vi "Actor Core.vi"(8 "error in":errorcluster, 11 "CS++DCPwrGui.lvclass":refnum<class "CS++FgenGui.lvclass">) -> (0 "Error Out":errorcluster, 3 "Actor out":refnum<class "Actor.lvclass">)   [LabVIEW 2015, in "CS++FgenGui.lvlib" / "CS++FgenGui.lvclass"]
doc: "(<B>Filename</B>: Actor Framework.lvlib:Actor.lvclass:Actor Core.vi)\n\nReceives messages to the actor, reacts to them, and initiates any error handling that may shut the actor down.\n\nDescendant classes may override this VI to append parallel tasks for the actor to complete while it handles messages. Overrides use the Call Parent Method node."
uses:
  CS++FgenGui.lvclass
  <vilib>/ActorFramework/Actor/Actor.lvclass
  CSPP_Core/Actors/CS++BaseActor/CS++BaseActor.lvclass/CS++BaseActor.ctl
  CSPP_Core/Actors/CS++GUIActor/CS++GUIActor.lvclass/CS++GUIActor.ctl
  CS++FgenChannelData/CS++FgenChannelData.lvclass
  <vilib>/ActorFramework/Actor/Actor.lvclass/Actor.ctl
  <vilib>/ActorFramework/Message Enqueuer/Message Enqueuer.lvclass/Message Enqueuer.ctl
  CSPP_Core/Classes/CS++ProcessVariables/ProcessVariable/PV.lvclass/PV.ctl
  CS++FgenChannelData/CS++FgenChannelData.lvclass/CS++FgenChannelData.ctl
  CSPP_Core/Actors/CS++BaseActor/Read Object Name.vi
  CSPP_Core/Actors/CS++BaseActor/Read CS++Factory.vi
  CSPP_Core/Actors/CS++GUIActor/Read Associated Actor Name.vi
  CSPP_Core/Classes/CS++ProcessVariables/ProcessVariable/Read Data.vi
  CSPP_Core/Classes/CS++ProcessVariables/ProcessVariable/Read Timestamp.vi
  CSPP_Core/Classes/CS++ProcessVariables/ProcessVariable/Read Name.vi
  CSPP_Core/Actors/CS++GUIActor/Read Stop-Event.vi
  CSPP_Core/Actors/CS++GUIActor/Read PV-Update.vi
  <vilib>/ActorFramework/Message Enqueuer/Init from Existing Queue.vi
  <vilib>/ActorFramework/Message Enqueuer/Enqueue.vi
  <vilib>/ActorFramework/Message Priority Queue/Priority Enqueue.vi
  CSPP_Core/Classes/CS++ProcessVariables/PVConnection/PVConnection.lvclass
  CSPP_Core/Classes/CS++BaseClasses/Factory/CS++Factory.lvclass
  CSPP_Core/Classes/CS++ProcessVariables/ProcessVariable/PV.lvclass
  <vilib>/ActorFramework/Message Enqueuer/Message Enqueuer.lvclass
  <vilib>/ActorFramework/Stop Msg/Stop Msg.lvclass
  CSPP_Core/Actors/CS++DeviceGUIActor/CS++DeviceGUIActor.lvclass
  CSPP_Core/Actors/CS++BaseActor/CS++BaseActor.lvclass
  CSPP_Core/Libraries/Utilities/CS++Utilities.lvlib
  CSPP_Core/Actors/CS++GUIActor/CS++GUIActor.lvclass
panel:
  in  "Tab Control":T1(tab)
  out "Associated Device Actor":string
  out "Driver Revision":string
  out "Firmware Revision":string
  out "Self-Test Result Code":i32
  out "Self-Test Result Message":string
  out "Resource Name":string
  out "Number Of Channels":i32
  out "Timestamp":timestamp
  in  "Tab Control 2":enum32{"General", "Channel"}(tab)
  in  "Sample Clock Output Enabled (Disabled)":bool caption="Sample Clock Output Enabled"
  in  "Sample Rate (1000 Samp/s)":dbl[unit]=1000.0 caption="Sample Rate" format="%.3e"
  in  "Internal Trigger Rate":dbl[unit] format="%^.3e"
  in  "Output Mode":i32(ring) items=["Standard Function", "Arbitrary Waveform", "Arbitrary Sequence"]
  in  "Reference Clock Source":i32(ring) caption="reference clock source (Internal)" items=["Internal"=0, "External"=1, "RTSI Clock"=101]
  in  "Sample Clock Source (Internal)":i32(ring) caption="Sample Clock Source" items=["Internal", "External"]
  in  "Config AM Modulation":bool
  in  "modulation frequency (1000 Hz)":dbl[unit]=1000.0 caption="AM Modulation Frequency" format="%^.2e"
  in  "modulation depth (0.00 %)":dbl caption="AM Modulation Depth /%" format="%.3f"
  in  "AM Modulation Waveform":i32(ring)=1 caption="modulation waveform (Sine)" items=["Sine"=1, "Square"=2, "Triangle"=3, "Ramp Up"=4, "Ramp Down"=5]
  in  "Config FM Modulation":bool
  in  "FM Modulation Frequency (1000 Hz)":dbl[unit]=1000.0 caption="FM Modulation Frequency" format="%^.2e"
  in  "FM Peak Deviation":dbl[unit]=100.0 format="%^.2e"
  in  "FM Modulation Waveform":i32(ring)=1 items=["Sine"=1, "Square"=2, "Triangle"=3, "Ramp Up"=4, "Ramp Down"=5]
  in  "Channel Index":i32 min=0 max=0 step=1
  in  "Tab Control 3":T2(tab)
  in  "Standard-Waveform":T3={"Enabled"=TRUE, "Operation Mode"=0, "Impedance"=50.0, "Waveform"=1, "Frequency"=1000.0, "Amplitude"=1.0, "DC Offset"=0.0, "Trigger Source"=1, "Burst Count"=1, "Start Phase"=0.0, "Set/Single"=FALSE} {"Start Phase" format="%.3f"; "Trigger Source" items=["Internal"=3, "External"=1, "Software Trigger Function"=2, "PXI TRIG0 or VXI TTL0"=111, "PXI TRIG1 or VXI TTL1"=112, "PXI TRIG2 or VXI TTL2"=113, "PXI TRIG3 or VXI TTL3"=114, "PXI TRIG4 or VXI TTL4"=115, "PXI TRIG5 or VXI TTL5"=116, "PXI TRIG6 or VXI TTL6"=117, "PXI TRIG7 or VXI TTL7"=118, "ECL0"=119, "ECL1"=120, "PXI Star"=131, "RTSI 0"=141, "RTSI 1"=142, "RTSI 2"=143, "RTSI 3"=144, "RTSI 4"=145, "RTSI 5"=146, "RTSI 6"=147]; "Frequency" format="%^.3e"; "DC Offset" format="%.3f"; "Amplitude" format="%.3f"; "Waveform" items=["Sine"=1, "Square"=2, "Triangle"=3, "Ramp Up"=4, "Ramp Down"=5, "DC"=6]; "Impedance" format="%.3f"; "Operation Mode" items=["Continuous", "Burst"]}
  in  "AM-Modulation":cluster{"Enabled":bool, "Source":i32}={"Enabled"=TRUE, "Source"=0} {"Source" items=["Internal", "External"]}
  in  "FM-Modulation":cluster{"Enabled":bool, "Source":i32}={"Enabled"=TRUE, "Source"=0} {"Source" items=["Internal", "External"]}
  in  "Advanced Trigger":T4 {"Trigger Slope)" items=["Positive", "Negative", "Either"]}
  in  "Start Trigger":T5 {"Trigger Slope" items=["Positive", "Negative", "Either"]}
  in  "Stop Trigger":T4 {"Trigger Slope)" items=["Positive", "Negative", "Either"]}
  in  "Resume Trigger":T4 {"Trigger Slope)" items=["Positive", "Negative", "Either"]}
  in  "Clear Arbitrary Waveform":bool
  in  "Clear Arbitrary Sequence":bool
  in  "Clear Arbitrary Memory":bool
  in  "SW Trigger":bool
  in  "SW Stop Trigger":bool
  in  "SW Resume Trigger":bool
  in  "SW Hold Trigger":bool
  in  "SW Advanced Trigger":bool
  in  "Initiate Generation":bool
  in  "Abort Generation":bool
  in  "Stop Button":bool
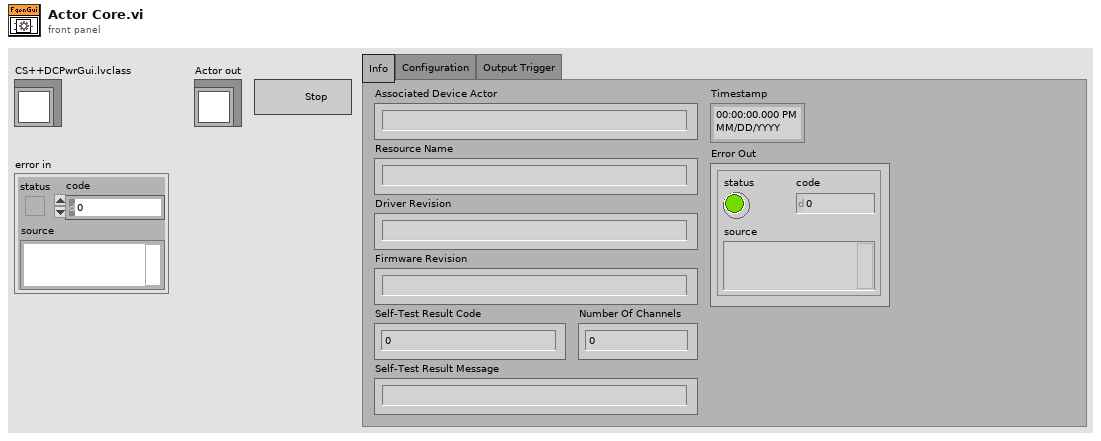
[diagram p1: front panel]
types:
  T1 = enum32{"Info", "Configuration", "Output Trigger"}
  T2 = enum32{"General", "AM/FM-Modulation", "More Trigger"}
  T3 = cluster{"Enabled":bool, "Operation Mode":i32, "Impedance":dbl[unit], "Waveform":i32, "Frequency":dbl[unit], "Amplitude":dbl[unit], "DC Offset":dbl[unit], "Trigger Source":i32, "Burst Count":i32, "Start Phase":dbl[unit], "Set/Single":bool}
  T4 = cluster{"Trigger Source":string, "Trigger Slope)":i32}
  T5 = cluster{"Trigger Source":string, "Trigger Slope":i32}
  T6 = enum32{"Invalid", "Standard", "Closed", "Hidden", "Minimized", "Maximized"}
  T7 = cluster{"AM Modulation Waveform":i32, "modulation depth (0.00 %)":dbl, "modulation frequency (1000 Hz)":dbl[unit]}
  T8 = cluster{"FM Modulation Waveform":i32, "FM Peak Deviation":dbl[unit], "FM Modulation Frequency (1000 Hz)":dbl[unit]}
  T9 = cluster{"Trigger Slope":i32, "Substring":string, "Trigger Source":string}
  T10 = cluster{"Trigger Slope)":i32, "Substring":string, "Trigger Source":string}
  T11 = cluster{"Start Phase":dbl[unit], "Frequency":dbl[unit], "DC Offset":dbl[unit], "Substring":string, "Amplitude":dbl[unit], "Waveform":i32}
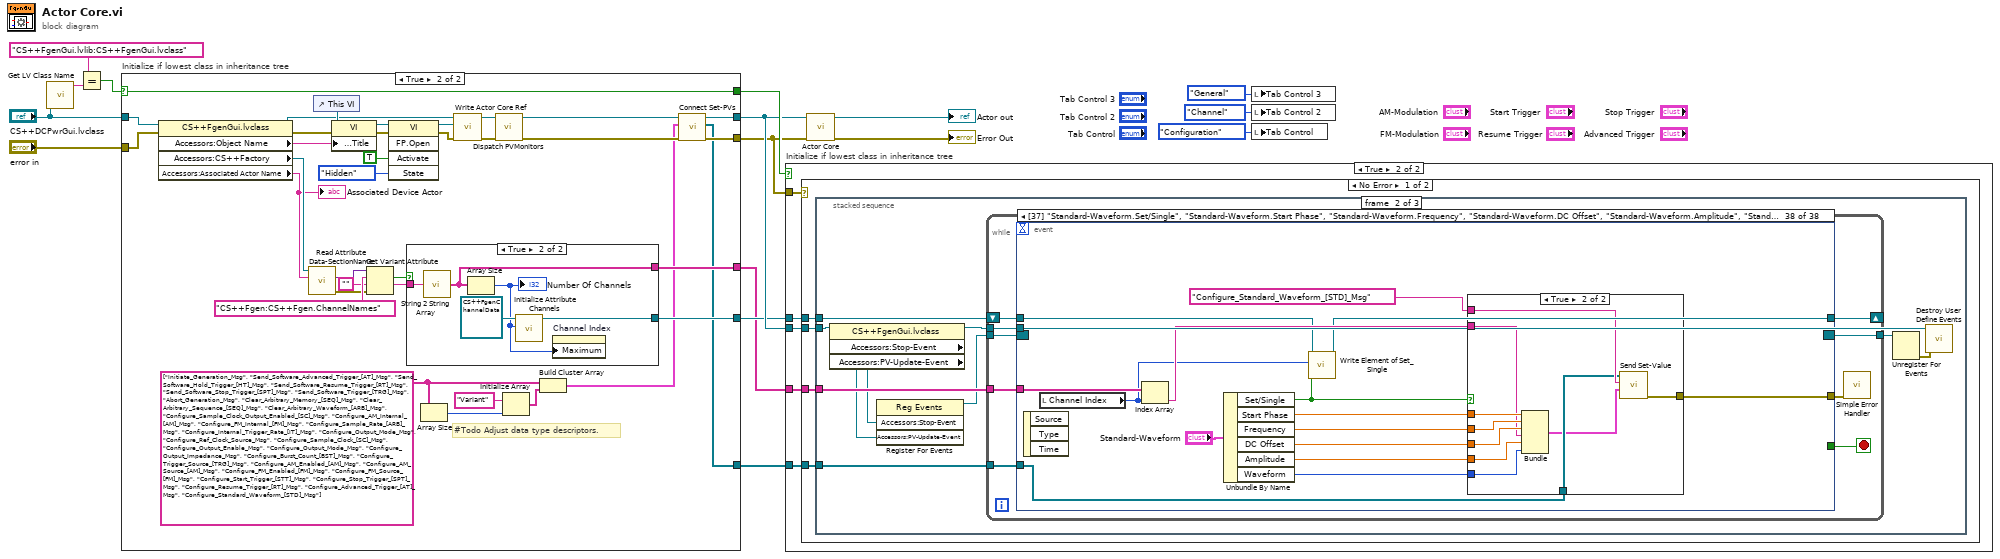
[diagram p0: block diagram]
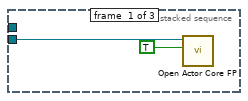
[diagram p5: hidden frame]
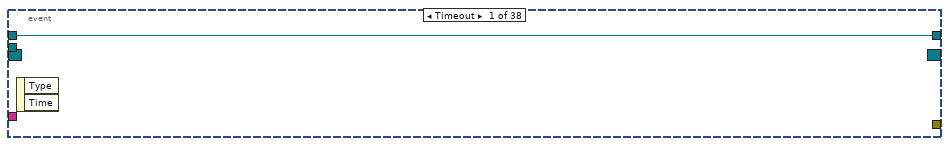
[diagram p6: hidden frame]
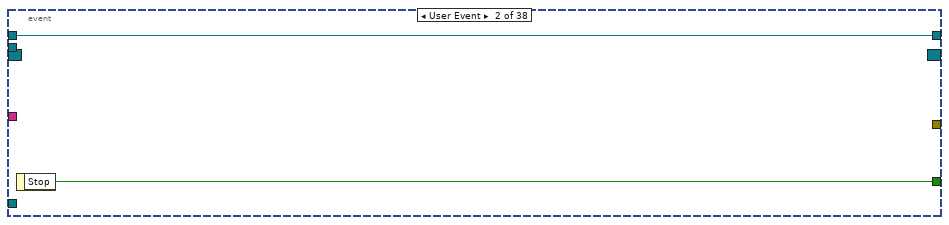
[diagram p7: hidden frame]
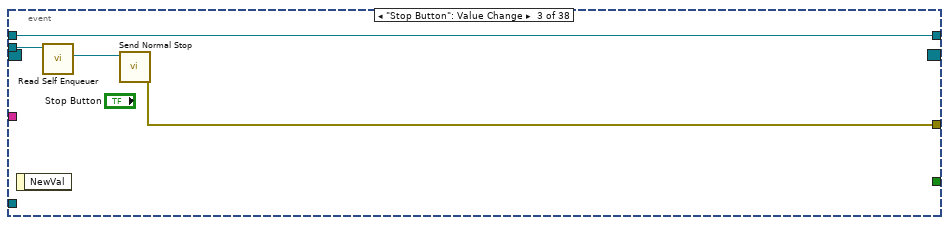
[diagram p8: hidden frame]
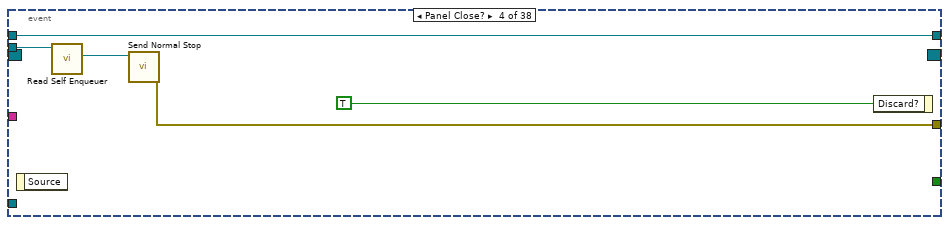
[diagram p9: hidden frame]
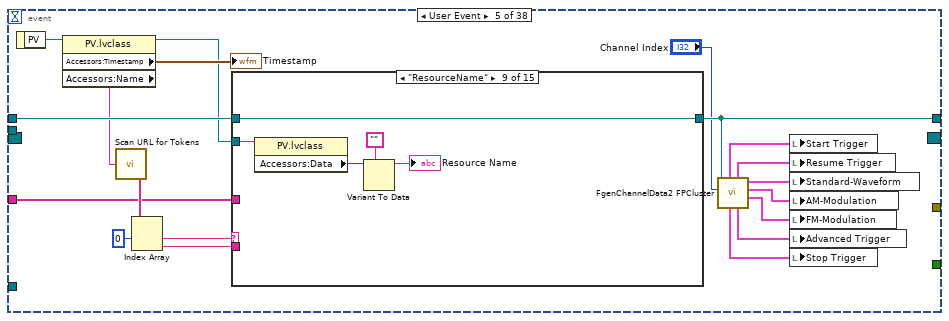
[diagram p10: hidden frame]
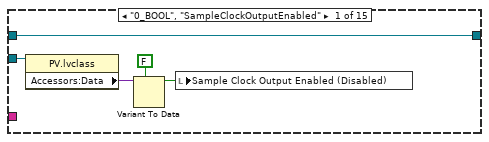
[diagram p11: hidden frame]
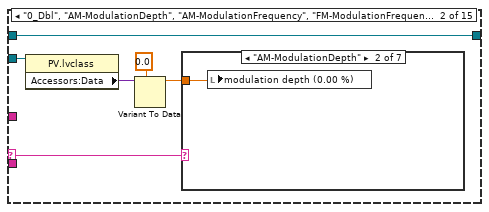
[diagram p12: hidden frame]
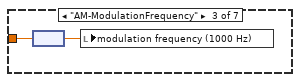
[diagram p14: hidden frame]
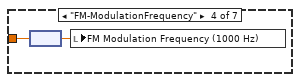
[diagram p15: hidden frame]
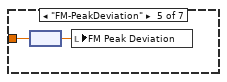
[diagram p16: hidden frame]
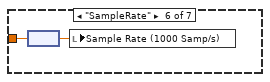
[diagram p17: hidden frame]
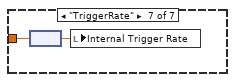
[diagram p18: hidden frame]
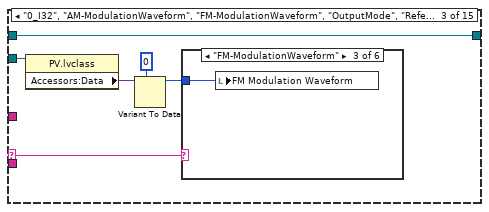
[diagram p19: hidden frame]
diagram:
  n1 = call <vilib>:"Get LV Class Name.vi"("object"="CS++DCPwrGui.lvclass") -> ("class name"=w14:string)  [unwired: 9 in, 1 out]
  n2 = Equal?(x="CS++FgenGui.lvlib:CS++FgenGui.lvclass" ("class name"), y=w14) -> (x = y?=w12:bool)
  n3 = case "Initialize if lowest class in inheritance tree" shown="True" w12 {
    selector: w12 -> [w17 w54]
    tunnel: [w18 w28] -> w7
    tunnel: "error in" -> [w18 w34]
    tunnel: [w19 w26] -> w8
    tunnel: "CS++DCPwrGui.lvclass" -> [w19 w35]
    tunnel: [w17 w54] -> w11
    tunnel: [_ w49] -> w6
    tunnel: [_ w48] -> w2
    tunnel: [_ w25] -> w1
    frame False {
    }
    frame True {
      w23 = string[] ["Initiate_Generation_Msg", "Send_Software_Advanced_Trigger_[AT]_Msg", "Send_Software_Hold_Trigger_[HT]_Msg", "Send_Software_Resume_Trigger_[RT]_Msg", "Send_Software_Stop_Trigger_[SPT]_Msg", "Send_Software_Trigger_[TRG]_Msg", "Abort_Generation_Msg", "Clear_Arbitrary_Memory_[SEQ]_Msg", "Clear_Arbitrary_Sequence_[SEQ]_Msg", "Clear_Arbitrary_Waveform_[ARB]_Msg", "Configure_Sample_Clock_Output_Enabled_[SC]_Msg", "Configure_AM_Internal_[AM]_Msg", "Configure_FM_Internal_[FM]_Msg", "Configure_Sample_Rate_[ARB]_Msg", "Configure_Internal_Trigger_Rate_[IT]_Msg", "Configure_Output_Mode_Msg", "Configure_Ref_Clock_Source_Msg", "Configure_Sample_Clock_[SC]_Msg", "Configure_Output_Enable_Msg", "Configure_Output_Mode_Msg", "Configure_Output_Impedance_Msg", "Configure_Burst_Count_[BST]_Msg", "Configure_Trigger_Source_[TRG]_Msg", "Configure_AM_Enabled_[AM]_Msg", "Configure_AM_Source_[AM]_Msg", "Configure_FM_Enabled_[FM]_Msg", "Configure_FM_Source_[FM]_Msg", "Configure_Start_Trigger_[STT]_Msg", "Configure_Stop_Trigger_[SPT]_Msg", "Configure_Resume_Trigger_[RT]_Msg", "Configure_Advanced_Trigger_[AT]_Msg", "Configure_Standard_Waveform_[STD]_Msg"]
      # "#Todo Adjust data type descriptors."
      n4 = property class="CS++FgenGui.lvclass"(reference=w35, error in=w34) -> (reference out=w39:refnum<class "CS++FgenGui.lvclass">, error out=w40:errorcluster, "Accessors:Object Name"=w38:string, "Accessors:CS++Factory"=w31:refnum<class "CS++Factory.lvclass">, "Accessors:Associated Actor Name"=w30:string)
      "Associated Device Actor" <- w30
      n5 = call-dynamic "Read Attribute Data-SectionName.vi"("Object Name"=w30, "CS++Factory in"=w31) -> ("error out"=w32:errorcluster, "Attribute Data"=w33:variant)  [unwired: 7 in, 1 out]
      n6 = control-ref of="This VI"() -> (w43:refnum<vi>)
      n7 = property class="VI"(reference=w43, error in=w40, "Front Panel.Title"=w38) -> (reference out=w42:refnum<vi>, error out=w41:errorcluster)
      n8 = Get Variant Attribute(Variant=w33, name="CS++Fgen:CS++Fgen.ChannelNames", default value (empty Variant)="", error in=w32) -> (found=w51:bool, value=w50:string)  [unwired: 2 out]
      n9 = invoke class="VI" method="FP.Open"(reference=w42, error in=w41, "Activate"=TRUE ("Activate?"), "State"=T6."Hidden") -> (reference out=w45:refnum<vi>, error out=w44:errorcluster)  [unwired: 1 in, 3 out]
      n10 = case shown="True" w51 {
        tunnel: w50 -> [_ w56]
        tunnel: [_ w58] -> w49
        tunnel: [_ w55] -> w48
        frame False {
        }
        frame True {
          n11 = call "String 2 String Array.vi"("String"=w56) -> ("Substrings"=w55:string[])  [unwired: 1 in]
          n12 = Array Size(array=w55) -> (size(s)=w57:i32)
          "Number Of Channels" <- w57
          n13 = call "Initialize Attribute Channels.vi"("Number of Channels"=w57, "CS++FgenChannelData in"=refnum<class "CS++FgenChannelData.lvclass"> refnum ("CS++FgenGui.lvlib:CS++FgenChannelData.lvclass")) -> ("CS++FgenChannelData out"=w58:refnum<class "CS++FgenChannelData.lvclass">)  [unwired: 8 in, 1 out]
          n14 = property on="Channel Index" class="DigNum (strict)"("Maximum"=w57) -> ()  [unwired: 2 in, 2 out]
        }
      }
      n15 = Array Size(array=w23) -> (size(s)=w22:i32)
      n16 = call "Write Actor Core Ref.vi"("error in (no error)"=w44, "Actor Core Ref"=w45, "CS++BaseActor in"=w39) -> ("error out"=w36:errorcluster, "CS++BaseActor out"=w37:refnum<class "CS++FgenGui.lvclass">)  [unwired: 7 in]
      n17 = call "Dispatch PVMonitors.vi"("Error In"=w36, "CS++GUIActor in"=w37) -> ("Error Out"=w29:errorcluster, "CS++GUIActor out"=w27:refnum<class "CS++FgenGui.lvclass">)  [unwired: 8 in]
      n18 = Initialize Array("Variant" ("element"), w22) -> (w20:string[])
      n19 = Build Cluster Array(w23, w20) -> (w24:cluster{string, "element":string}[])
      n20 = call "Connect Set-PVs.vi"("Error In"=w29, "Set-Messages"=w24, "CS++GUIActor in"=w27) -> ("Error Out"=w28:errorcluster, "PVConnections"=w25:refnum<class "PVConnection.lvclass">[], "CS++GUIActor out"=w26:refnum<class "CS++FgenGui.lvclass">)  [unwired: 6 in]
    }
  }
  n21 = case "Initialize if lowest class in inheritance tree" shown="True" w11 {
    tunnel: w7 -> [_ w64]
    tunnel: w8 -> [_ w63]
    tunnel: w6 -> [_ w62]
    tunnel: w2 -> [_ w61]
    tunnel: w1 -> [_ w60]
    frame False {
    }
    frame True {
      n22 = case shown="No Error" w64 {
        tunnel: w63 -> [w68 _]
        tunnel: w62 -> [w67 _]
        tunnel: w61 -> [w66 _]
        tunnel: w60 -> [w65 _]
        frame No Error {
          n23 = stacked-sequence {
            tunnel: w68 -> [w70 w76 w622]
            tunnel: w67 -> [_ w80 _]
            tunnel: w66 -> [_ w79 _]
            tunnel: w65 -> [_ w71 w620]
            frame #0 {
              n24 = call "Open Actor Core FP.vi"("Open FP (F)"=TRUE, "CS++BaseActor in"=w70) -> ()  [unwired: 8 in, 2 out]
            }
            frame #1 {
              n25 = property class="CS++FgenGui.lvclass"(reference=w76) -> (reference out=w75:refnum<class "CS++FgenGui.lvclass">, "Accessors:Stop-Event"=w73:refnum<user-event>, "Accessors:PV-Update-Event"=w72:refnum<user-event>)  [unwired: 1 in, 1 out]
              n26 = register-events(w73, w72) -> (reference out=w74:refnum<event-registration>)  [unwired: 2 in, 1 out]
              n27 = while {
                tunnel: w74 -> [w89]
                tunnel: w75 -> [w88]
                tunnel: [w86] -> w78
                shift-right: [w83] -> _
                shift-left: w80 -> [w84]
                tunnel: w79 -> [w82]
                tunnel: w71 -> [w81]
                stop <- w87 stop-if-true
                n28 = event shown="[37] \"Standard-Waveform.Set/Single\", \"Standard-Waveform.Start Phase\", \"Standard-Waveform.Frequency\", \"Standard-Waveform.DC Offset\", \"Standard-Waveform.Amplitude\", \"Standard-Waveform.Waveform\": Value Change" {
                  selector: w89 -> [_ _ _ _ _ _ _ _ _ _ _ _ _ _ _ _ _ _ _ _ _ _ _ _ _ _ _ _ _ _ _ _ _ _ _ _ _ _]
                  dyn-events: [_ _ _ _ _ _ _ _ _ _ _ _ _ _ _ _ _ _ _ _ _ _ _ _ _ _ _ _ _ _ _ _ _ _ _ _ _ _] -> w86
                  timeout: _ -> [_ _ _ _ _ _ _ _ _ _ _ _ _ _ _ _ _ _ _ _ _ _ _ _ _ _ _ _ _ _ _ _ _ _ _ _ _ _]
                  tunnel: w88 -> [_ _ w96 w99 _ _ _ _ _ _ _ _ _ _ _ _ _ _ _ _ _ _ _ _ _ _ _ _ _ _ _ _ _ _ _ _ _ _]
                  tunnel: [_ w92 _ _ _ _ _ _ _ _ _ _ _ _ _ _ _ _ _ _ _ _ _ _ _ _ _ _ _ _ _ _ _ _ _ _ _ _] -> w87
                  tunnel: [_ _ w94 w98 _ w336 w347 w355 w363 w371 w379 w387 w395 w403 w411 w419 w424 w429 w441 w447 w453 w458 w463 w468 w475 w484 w493 w502 w511 w520 w529 w538 w547 w557 w568 w579 w590 w607] -> w85
                  tunnel: w84 -> [w90 w91 w93 w97 w114 w342 w345 w353 w361 w369 w377 w385 w393 w401 w409 w417 w428 w436 w444 w449 w454 w459 w464 w469 w478 w487 w496 w505 w514 w523 w532 w541 w550 w561 w572 w583 w594 w600]
                  tunnel: [w90 w91 w93 w97 w106 w342 w345 w353 w361 w369 w377 w385 w393 w401 w409 w417 w428 w436 w444 w449 w454 w459 w464 w469 w478 w487 w496 w505 w514 w523 w532 w541 w550 w561 w572 w583 w594 w599] -> w83
                  tunnel: w82 -> [_ _ _ _ w104 _ _ _ _ _ _ _ _ _ _ _ _ _ _ _ _ _ _ _ w477 w486 w495 w504 w513 w522 w531 w540 w549 w560 w571 w582 w593 w609]
                  tunnel: w81 -> [_ _ _ _ _ _ w344 w352 w360 w368 w376 w384 w392 w400 w408 w416 w426 w434 w442 w446 w452 w456 w461 w466 w473 w483 w491 w500 w510 w519 w527 w536 w546 w555 w567 w578 w588 w595]
                  event Timeout {
                    n29 = event-data() -> ()  [unwired: 1 in, 2 out]
                  }
                  event User Event {
                    n30 = event-data() -> ("Stop"=w92:bool)  [unwired: 1 in]
                  }
                  event "Stop Button": Value Change {
                    n31 = event-data() -> ()  [unwired: 1 in, 1 out]
                    n32 = call <vilib>:"Read Self Enqueuer.vi"("Actor"=w96) -> ("Self Enqueuer"=w95:refnum<class "Message Enqueuer.lvclass">)  [unwired: 10 in]
                    n33 = call <vilib>:"Send Normal Stop.vi"("Message Enqueuer"=w95) -> ("error out"=w94:errorcluster)  [unwired: 10 in]
                  }
                  event Panel Close? {
                    n34 = event-data() -> ()  [unwired: 1 in, 1 out]
                    n35 = call <vilib>:"Read Self Enqueuer.vi"("Actor"=w99) -> ("Self Enqueuer"=w100:refnum<class "Message Enqueuer.lvclass">)  [unwired: 10 in]
                    n36 = call <vilib>:"Send Normal Stop.vi"("Message Enqueuer"=w100) -> ("error out"=w98:errorcluster)  [unwired: 10 in]
                    n37 = event-data("Discard?"=TRUE) -> ()  [unwired: 1 in, 1 out]
                  }
                  event User Event {
                    n38 = event-data() -> ("PV"=w117:refnum<class "PV.lvclass">)  [unwired: 1 in]
                    n39 = property class="PV.lvclass"(reference=w117) -> (reference out=w102:refnum<class "PV.lvclass">, "Accessors:Timestamp"=→"Timestamp":timestamp, "Accessors:Name"=w103:string)  [unwired: 1 in, 1 out]
                    n40 = call "Scan URL for Tokens.vi"("URL"=w103) -> ("Tokens"=w120:string[])
                    n41 = Index Array(array=w120, index #1=0 ("index")) -> (element #1=w115:string, element #2=w118:string)  [unwired: 1 in]
                    n42 = case shown="\"ResourceName\"" w115 {
                      selector: w115 -> [_ w128 w145 w160 w183 w234 w275 _ _ _ _ _ _ _ _]
                      tunnel: w102 -> [w125 w129 w146 w161 w184 w235 w277 _ w298 w303 w308 w314 w319 w324 w330]
                      tunnel: w118 -> [_ _ _ w155 w178 w229 w270 _ _ _ _ _ _ _ _]
                      tunnel: [w121 w126 w143 w159 w182 w233 w274 w296 w301 w306 w311 w317 w322 w327 w333] -> w106
                      tunnel: w114 -> [w121 w126 w143 w158 w181 w232 w273 w296 w301 w306 w311 w317 w322 w327 w333]
                      tunnel: w104 -> [_ _ _ w156 w179 w230 w271 _ _ _ _ _ _ _ _]
                      frame "0_BOOL", "SampleClockOutputEnabled" {
                        n43 = property class="PV.lvclass"(reference=w125) -> ("Accessors:Data"=w123:variant)  [unwired: 1 in, 2 out]
                        n44 = Variant To Data(type=FALSE, Variant=w123) -> (data=w122:bool)  [unwired: 1 in, 1 out]
                        n45 = local write "Sample Clock Output Enabled (Disabled)"(w122) -> ()
                      }
                      frame "0_Dbl", "AM-ModulationDepth", "AM-ModulationFrequency", "FM-ModulationFrequency", "FM-PeakDeviation", "SampleRate", "TriggerRate" {
                        n46 = property class="PV.lvclass"(reference=w129) -> ("Accessors:Data"=w130:variant)  [unwired: 1 in, 2 out]
                        n47 = Variant To Data(type=0.0, Variant=w130) -> (data=w127:dbl)  [unwired: 1 in, 1 out]
                        n48 = case shown="\"AM-ModulationDepth\"" w128 {
                          tunnel: w127 -> [_ w132 w134 w136 w138 w140 w142]
                          frame Default {
                          }
                          frame "AM-ModulationDepth" {
                            n49 = local write "modulation depth (0.00 %)"(w132) -> ()
                          }
                          frame "AM-ModulationFrequency" {
                            n50 = node(w134) -> (w133:dbl[unit])
                            n51 = local write "modulation frequency (1000 Hz)"(w133) -> ()
                          }
                          frame "FM-ModulationFrequency" {
                            n52 = node(w136) -> (w135:dbl[unit])
                            n53 = local write "FM Modulation Frequency (1000 Hz)"(w135) -> ()
                          }
                          frame "FM-PeakDeviation" {
                            n54 = node(w138) -> (w137:dbl[unit])
                            n55 = local write "FM Peak Deviation"(w137) -> ()
                          }
                          frame "SampleRate" {
                            n56 = node(w140) -> (w139:dbl[unit])
                            n57 = local write "Sample Rate (1000 Samp/s)"(w139) -> ()
                          }
                          frame "TriggerRate" {
                            n58 = node(w142) -> (w141:dbl[unit])
                            n59 = local write "Internal Trigger Rate"(w141) -> ()
                          }
                        }
                      }
                      frame "0_I32", "AM-ModulationWaveform", "FM-ModulationWaveform", "OutputMode", "ReferenceClockSource", "SampleClockSource" {
                        n60 = property class="PV.lvclass"(reference=w146) -> ("Accessors:Data"=w147:variant)  [unwired: 1 in, 2 out]
                        n61 = Variant To Data(type=0, Variant=w147) -> (data=w144:i32)  [unwired: 1 in, 1 out]
                        n62 = case shown="\"FM-ModulationWaveform\"" w145 {
                          tunnel: w144 -> [_ w149 w150 w151 w152 w153]
                          frame Default {
                          }
                          frame "AM-ModulationWaveform" {
                            n63 = local write "AM Modulation Waveform"(w149) -> ()
                          }
                          frame "FM-ModulationWaveform" {
                            n64 = local write "FM Modulation Waveform"(w150) -> ()
                          }
                          frame "OutputMode" {
                            n65 = local write "Output Mode"(w151) -> ()
                          }
                          frame "ReferenceClockSource" {
                            n66 = local write "Reference Clock Source"(w152) -> ()
                          }
                          frame "SampleClockSource" {
                            n67 = local write "Sample Clock Source (Internal)"(w153) -> ()
                          }
                        }
                      }
                      frame "0_[Bool]", "AM-Enabled", "ChannelEnabled", "FM-Enabled" {
                        n68 = property class="PV.lvclass"(reference=w161) -> ("Accessors:Data"=w162:variant)  [unwired: 1 in, 2 out]
                        n69 = Search 1D Array(1D array=w156, element=w155) -> (index of element=w154:i32)  [unwired: 1 in]
                        n70 = Variant To Data(type=FALSE, Variant=w162) -> (data=w157:bool)  [unwired: 1 in, 1 out]
                        n71 = case shown="\"AM-Enabled\"" w160 {
                          tunnel: [w164 w167 w171 w175] -> w159
                          tunnel: w158 -> [w164 w168 w172 w176]
                          tunnel: w154 -> [_ w166 w170 w173]
                          tunnel: w157 -> [_ w165 w169 w174]
                          frame Default {
                          }
                          frame "AM-Enabled" {
                            n72 = call "Write Element of AM Enabled.vi"("AM enabled (True)"=w165, "index"=w166, "CS++FgenChannelData in"=w168) -> ("CS++FgenChannelData out"=w167:refnum<class "CS++FgenChannelData.lvclass">)  [unwired: 7 in, 1 out]
                          }
                          frame "ChannelEnabled" {
                            n73 = call "Write Element of Channel Enabled.vi"("channel enabled (True)"=w169, "index"=w170, "CS++FgenChannelData in"=w172) -> ("CS++FgenChannelData out"=w171:refnum<class "CS++FgenChannelData.lvclass">)  [unwired: 7 in, 1 out]
                          }
                          frame "FM-Enabled" {
                            n74 = call "Write Element of FM enabled.vi"("FM enabled (True)"=w174, "index"=w173, "CS++FgenChannelData in"=w176) -> ("CS++FgenChannelData out"=w175:refnum<class "CS++FgenChannelData.lvclass">)  [unwired: 7 in, 1 out]
                          }
                        }
                      }
                      frame "0_[I32]", "AM-Source", "AdvancedTriggerSlope", "BurstCount", "FM-Source", "OperationMode", "ResumeTriggerSlope", "StartTriggerSlope", "StopTriggerSlope", "TriggerSource", "Waveform" {
                        n75 = property class="PV.lvclass"(reference=w184) -> ("Accessors:Data"=w185:variant)  [unwired: 1 in, 2 out]
                        n76 = Search 1D Array(1D array=w179, element=w178) -> (index of element=w177:i32)  [unwired: 1 in]
                        n77 = Variant To Data(type=0, Variant=w185) -> (data=w180:i32)  [unwired: 1 in, 1 out]
                        n78 = case shown="\"AM-Source\"" w183 {
                          tunnel: [w187 w188 w194 w198 w202 w206 w208 w214 w218 w222 w226] -> w182
                          tunnel: w181 -> [w187 w191 w195 w199 w203 w207 w211 w215 w219 w223 w227]
                          tunnel: w177 -> [_ w190 w193 w197 w201 w204 w209 w213 w217 w221 w225]
                          tunnel: w180 -> [_ w189 w192 w196 w200 w205 w210 w212 w216 w220 w224]
                          frame Default {
                          }
                          frame "AM-Source" {
                            n79 = call "Write Element of AM Source.vi"("source (Internal)"=w189, "index"=w190, "CS++FgenChannelData in"=w191) -> ("CS++FgenChannelData out"=w188:refnum<class "CS++FgenChannelData.lvclass">)  [unwired: 7 in, 1 out]
                          }
                          frame "AdvancedTriggerSlope" {
                            n80 = call "Write Element of Advanced Trigger Slope.vi"("Trigger Slope (Positive)"=w192, "index"=w193, "CS++FgenChannelData in"=w195) -> ("CS++FgenChannelData out"=w194:refnum<class "CS++FgenChannelData.lvclass">)  [unwired: 7 in, 1 out]
                          }
                          frame "BurstCount" {
                            n81 = call "Write Element of Burst Count.vi"("burst count (1)"=w196, "index"=w197, "CS++FgenChannelData in"=w199) -> ("CS++FgenChannelData out"=w198:refnum<class "CS++FgenChannelData.lvclass">)  [unwired: 7 in, 1 out]
                          }
                          frame "FM-Source" {
                            n82 = call "Write Element of FM Source.vi"("source (Internal)"=w200, "index"=w201, "CS++FgenChannelData in"=w203) -> ("CS++FgenChannelData out"=w202:refnum<class "CS++FgenChannelData.lvclass">)  [unwired: 7 in, 1 out]
                          }
                          frame "OperationMode" {
                            n83 = call "Write Element of Operation Mode.vi"("operation mode (Continuous)"=w205, "index"=w204, "CS++FgenChannelData in"=w207) -> ("CS++FgenChannelData out"=w206:refnum<class "CS++FgenChannelData.lvclass">)  [unwired: 7 in, 1 out]
                          }
                          frame "ResumeTriggerSlope" {
                            n84 = call "Write Element of Resume Trigger Slope.vi"("Trigger Slope (Positive)"=w210, "index"=w209, "CS++FgenChannelData in"=w211) -> ("CS++FgenChannelData out"=w208:refnum<class "CS++FgenChannelData.lvclass">)  [unwired: 7 in, 1 out]
                          }
                          frame "StartTriggerSlope" {
                            n85 = call "Write Element of Start Trigger Slope.vi"("Trigger Slope (Positive)"=w212, "index"=w213, "CS++FgenChannelData in"=w215) -> ("CS++FgenChannelData out"=w214:refnum<class "CS++FgenChannelData.lvclass">)  [unwired: 7 in, 1 out]
                          }
                          frame "StopTriggerSlope" {
                            n86 = call "Write Element of Stop Trigger Slope.vi"("Trigger Slope (Positive)"=w216, "index"=w217, "CS++FgenChannelData in"=w219) -> ("CS++FgenChannelData out"=w218:refnum<class "CS++FgenChannelData.lvclass">)  [unwired: 7 in, 1 out]
                          }
                          frame "TriggerSource" {
                            n87 = call "Write Element of Trigger Source.vi"("trigger source (External)"=w220, "index"=w221, "CS++FgenChannelData in"=w223) -> ("CS++FgenChannelData out"=w222:refnum<class "CS++FgenChannelData.lvclass">)  [unwired: 7 in, 1 out]
                          }
                          frame "Waveform" {
                            n88 = call "Write Element of Waveform.vi"("waveform (Sine)"=w224, "index"=w225, "CS++FgenChannelData in"=w227) -> ("CS++FgenChannelData out"=w226:refnum<class "CS++FgenChannelData.lvclass">)  [unwired: 7 in, 1 out]
                          }
                        }
                      }
                      frame "0_[Dbl]", "Amplitude", "Arb-Frequency", "DCOffset", "Frequency", "OutputImpedance", "StartPhase" {
                        n89 = property class="PV.lvclass"(reference=w235) -> ("Accessors:Data"=w236:variant)  [unwired: 1 in, 2 out]
                        n90 = Search 1D Array(1D array=w230, element=w229) -> (index of element=w228:i32)  [unwired: 1 in]
                        n91 = Variant To Data(type=0.0, Variant=w236) -> (data=w231:dbl)  [unwired: 1 in, 1 out]
                        n92 = case shown="\"Amplitude\"" w234 {
                          tunnel: [w238 w242 w247 w251 w254 w262 w267] -> w233
                          tunnel: w232 -> [w238 w243 w248 w252 w258 w263 w268]
                          tunnel: w228 -> [_ w241 w246 w249 w255 w259 w264]
                          tunnel: w231 -> [_ w240 w245 w253 w257 w261 w266]
                          frame Default {
                          }
                          frame "Amplitude" {
                            n93 = node(w240) -> (w239:dbl[unit])
                            n94 = call "Write Element of Amplitude.vi"("amplitude (1.00 V)"=w239, "index"=w241, "CS++FgenChannelData in"=w243) -> ("CS++FgenChannelData out"=w242:refnum<class "CS++FgenChannelData.lvclass">)  [unwired: 7 in, 1 out]
                          }
                          frame "Arb-Frequency" {
                            n95 = node(w245) -> (w244:dbl[unit])
                            n96 = call "Write Element of Arb Frequency.vi"("frequency (0.0 Hz)"=w244, "index"=w246, "CS++FgenChannelData in"=w248) -> ("CS++FgenChannelData out"=w247:refnum<class "CS++FgenChannelData.lvclass">)  [unwired: 7 in, 1 out]
                          }
                          frame "DCOffset" {
                            n97 = node(w253) -> (w250:dbl[unit])
                            n98 = call "Write Element of DC Offset.vi"("dc offset (0.00 V)"=w250, "index"=w249, "CS++FgenChannelData in"=w252) -> ("CS++FgenChannelData out"=w251:refnum<class "CS++FgenChannelData.lvclass">)  [unwired: 7 in, 1 out]
                          }
                          frame "Frequency" {
                            n99 = node(w257) -> (w256:dbl[unit])
                            n100 = call "Write Element of Frequency.vi"("frequency (1000.0 Hz)"=w256, "index"=w255, "CS++FgenChannelData in"=w258) -> ("CS++FgenChannelData out"=w254:refnum<class "CS++FgenChannelData.lvclass">)  [unwired: 7 in, 1 out]
                          }
                          frame "OutputImpedance" {
                            n101 = node(w261) -> (w260:dbl[unit])
                            n102 = call "Write Element of Output Impedance.vi"("impedance (50 Ohms)"=w260, "index"=w259, "CS++FgenChannelData in"=w263) -> ("CS++FgenChannelData out"=w262:refnum<class "CS++FgenChannelData.lvclass">)  [unwired: 7 in, 1 out]
                          }
                          frame "StartPhase" {
                            n103 = node(w266) -> (w265:dbl[unit])
                            n104 = call "Write Element of Start Phase.vi"("start phase (0.00 Degrees)"=w265, "index"=w264, "CS++FgenChannelData in"=w268) -> ("CS++FgenChannelData out"=w267:refnum<class "CS++FgenChannelData.lvclass">)  [unwired: 7 in, 1 out]
                          }
                        }
                      }
                      frame "0_[Str]", "AdvancedTriggerSource", "ResumeTriggerSource", "StartTriggerSource", "StopTriggerSource" {
                        n105 = property class="PV.lvclass"(reference=w277) -> ("Accessors:Data"=w278:variant)  [unwired: 1 in, 2 out]
                        n106 = Search 1D Array(1D array=w271, element=w270) -> (index of element=w269:i32)  [unwired: 1 in]
                        n107 = Variant To Data(type="", Variant=w278) -> (data=w272:string)  [unwired: 1 in, 1 out]
                        n108 = case shown="\"ResumeTriggerSource\"" w275 {
                          tunnel: [w279 w280 w286 w290 w294] -> w274
                          tunnel: w273 -> [w279 w283 w287 w291 w295]
                          tunnel: w272 -> [_ w282 w284 w288 w292]
                          tunnel: w269 -> [_ w281 w285 w289 w293]
                          frame Default {
                          }
                          frame "AdvancedTriggerSource" {
                            n109 = call "Write Element of Advanced Trigger Source.vi"("Trigger Source (None)"=w282, "index"=w281, "CS++FgenChannelData in"=w283) -> ("CS++FgenChannelData out"=w280:refnum<class "CS++FgenChannelData.lvclass">)  [unwired: 7 in, 1 out]
                          }
                          frame "ResumeTriggerSource" {
                            n110 = call "Write Element of Resume Trigger Source.vi"("Trigger Source (None)"=w284, "index"=w285, "CS++FgenChannelData in"=w287) -> ("CS++FgenChannelData out"=w286:refnum<class "CS++FgenChannelData.lvclass">)  [unwired: 7 in, 1 out]
                          }
                          frame "StartTriggerSource" {
                            n111 = call "Write Element of Start Trigger Source.vi"("Trigger Source (None)"=w288, "index"=w289, "CS++FgenChannelData in"=w291) -> ("CS++FgenChannelData out"=w290:refnum<class "CS++FgenChannelData.lvclass">)  [unwired: 7 in, 1 out]
                          }
                          frame "StopTriggerSource" {
                            n112 = call "Write Element of Stop Trigger Source.vi"("Trigger Source (None)"=w292, "index"=w293, "CS++FgenChannelData in"=w295) -> ("CS++FgenChannelData out"=w294:refnum<class "CS++FgenChannelData.lvclass">)  [unwired: 7 in, 1 out]
                          }
                        }
                      }
                      frame Default {
                      }
                      frame "ResourceName" {
                        n113 = property class="PV.lvclass"(reference=w298) -> ("Accessors:Data"=w300:variant)  [unwired: 1 in, 2 out]
                        n114 = Variant To Data(type="", Variant=w300) -> (data=→"Resource Name":string)  [unwired: 1 in, 1 out]
                      }
                      frame "DriverRevision" {
                        n115 = property class="PV.lvclass"(reference=w303) -> ("Accessors:Data"=w305:variant)  [unwired: 1 in, 2 out]
                        n116 = Variant To Data(type="", Variant=w305) -> (data=→"Driver Revision":string)  [unwired: 1 in, 1 out]
                      }
                      frame "FirmwareRevision" {
                        n117 = property class="PV.lvclass"(reference=w308) -> ("Accessors:Data"=w310:variant)  [unwired: 1 in, 2 out]
                        n118 = Variant To Data(type="", Variant=w310) -> (data=→"Firmware Revision":string)  [unwired: 1 in, 1 out]
                      }
                      frame "ErrorMessage" {
                        n119 = property class="PV.lvclass"(reference=w314) -> ("Accessors:Data"=w316:variant)  [unwired: 1 in, 2 out]
                        n120 = Variant To Data(type="", Variant=w316) -> (data=w313:string, error out=w312:errorcluster)  [unwired: 1 in]
                        n121 = property on="source" class="Str"(error in=w312, "Value"=w313) -> ()  [unwired: 1 in, 2 out]
                      }
                      frame "SelftestResultMessage" {
                        n122 = property class="PV.lvclass"(reference=w319) -> ("Accessors:Data"=w321:variant)  [unwired: 1 in, 2 out]
                        n123 = Variant To Data(type="", Variant=w321) -> (data=→"Self-Test Result Message":string)  [unwired: 1 in, 1 out]
                      }
                      frame "SelftestResultCode" {
                        n124 = property class="PV.lvclass"(reference=w324) -> ("Accessors:Data"=w326:variant)  [unwired: 1 in, 2 out]
                        n125 = Variant To Data(type=0, Variant=w326) -> (data=→"Self-Test Result Code":i32)  [unwired: 1 in, 1 out]
                      }
                      frame "ErrorCode" {
                        n126 = property class="PV.lvclass"(reference=w330) -> ("Accessors:Data"=w332:variant)  [unwired: 1 in, 2 out]
                        n127 = Variant To Data(type=0, Variant=w332) -> (data=w328:i32, error out=w329:errorcluster)  [unwired: 1 in]
                        n128 = property on="code" class="DigNum (strict)"(error in=w329, "Value"=w328) -> ()  [unwired: 1 in, 2 out]
                      }
                    }
                    n129 = call "FgenChannelData2 FPCluster.vi"("Channel Index"="Channel Index", "CS++FgenChannelData in"=w106) -> ("FM-Modulation"=w109:cluster{"Enabled":bool, "Source":i32}, "AM-Modulation"=w110:cluster{"Enabled":bool, "Source":i32}, "Standard-Waveform"=w113:T3, "Advanced Trigger"=w108:T4, "Resume Trigger"=w112:T4, "Stop Trigger"=w107:T4, "Start Trigger"=w111:T4)  [unwired: 2 in, 1 out]
                    n130 = local write "Start Trigger"(w111) -> ()
                    n131 = local write "Resume Trigger"(w112) -> ()
                    n132 = local write "Standard-Waveform"(w113) -> ()
                    n133 = local write "AM-Modulation"(w110) -> ()
                    n134 = local write "FM-Modulation"(w109) -> ()
                    n135 = local write "Advanced Trigger"(w108) -> ()
                    n136 = local write "Stop Trigger"(w107) -> ()
                  }
                  event "Channel Index": Value Change {
                    n137 = event-data() -> ("NewVal"=w343:i32)  [unwired: 1 in]
                    n138 = call "FgenChannelData2 FPCluster.vi"("Channel Index"=w343, "CS++FgenChannelData in"=w342) -> ("error out"=w336:errorcluster, "FM-Modulation"=w337:cluster{"Enabled":bool, "Source":i32}, "AM-Modulation"=w338:cluster{"Enabled":bool, "Source":i32}, "Standard-Waveform"=w341:T3, "Advanced Trigger"=w335:T4, "Resume Trigger"=w340:T4, "Stop Trigger"=w334:T4, "Start Trigger"=w339:T4)  [unwired: 2 in]
                    n139 = local write "Start Trigger"(w339) -> ()
                    n140 = local write "Resume Trigger"(w340) -> ()
                    n141 = local write "Standard-Waveform"(w341) -> ()
                    n142 = local write "AM-Modulation"(w338) -> ()
                    n143 = local write "FM-Modulation"(w337) -> ()
                    n144 = local write "Advanced Trigger"(w335) -> ()
                    n145 = local write "Stop Trigger"(w334) -> ()
                  }
                  event "Initiate Generation": Value Change {
                    n146 = event-data() -> ("NewVal"=w346:bool)  [unwired: 1 in]
                    n147 = case shown="True" w346 {
                      tunnel: [_ w350] -> w347
                      tunnel: w344 -> [_ w349]
                      frame False {
                      }
                      frame True {
                        n148 = call "Send Msg Trigger.vi"("Trigger Msg (F)"=TRUE, "PVName"="Initiate_Acquisition_Msg", "PVConnections"=w349) -> ("error out"=w350:errorcluster)  [unwired: 7 in, 1 out]
                      }
                    }
                  }
                  event "SW Advanced Trigger": Value Change {
                    n149 = event-data() -> ("NewVal"=w354:bool)  [unwired: 1 in]
                    n150 = case shown="True" w354 {
                      tunnel: [_ w359] -> w355
                      tunnel: w352 -> [_ w357]
                      frame False {
                      }
                      frame True {
                        n151 = call "Send Msg Trigger.vi"("Trigger Msg (F)"=TRUE, "PVName"="Send_Software_Advanced_Trigger_[AT]_Msg", "PVConnections"=w357) -> ("error out"=w359:errorcluster)  [unwired: 7 in, 1 out]
                      }
                    }
                  }
                  event "SW Hold Trigger": Value Change {
                    n152 = event-data() -> ("NewVal"=w362:bool)  [unwired: 1 in]
                    n153 = case shown="True" w362 {
                      tunnel: [_ w367] -> w363
                      tunnel: w360 -> [_ w365]
                      frame False {
                      }
                      frame True {
                        n154 = call "Send Msg Trigger.vi"("Trigger Msg (F)"=TRUE, "PVName"="Send_Software_Hold_Trigger_[HT]_Msg", "PVConnections"=w365) -> ("error out"=w367:errorcluster)  [unwired: 7 in, 1 out]
                      }
                    }
                  }
                  event "SW Resume Trigger": Value Change {
                    n155 = event-data() -> ("NewVal"=w370:bool)  [unwired: 1 in]
                    n156 = case shown="True" w370 {
                      tunnel: [_ w375] -> w371
                      tunnel: w368 -> [_ w373]
                      frame False {
                      }
                      frame True {
                        n157 = call "Send Msg Trigger.vi"("Trigger Msg (F)"=TRUE, "PVName"="Send_Software_Resume_Trigger_[RT]_Msg", "PVConnections"=w373) -> ("error out"=w375:errorcluster)  [unwired: 7 in, 1 out]
                      }
                    }
                  }
                  event "SW Stop Trigger": Value Change {
                    n158 = event-data() -> ("NewVal"=w378:bool)  [unwired: 1 in]
                    n159 = case shown="True" w378 {
                      tunnel: [_ w383] -> w379
                      tunnel: w376 -> [_ w382]
                      frame False {
                      }
                      frame True {
                        n160 = call "Send Msg Trigger.vi"("Trigger Msg (F)"=TRUE, "PVName"="Send_Software_Stop_Trigger_[SPT]_Msg", "PVConnections"=w382) -> ("error out"=w383:errorcluster)  [unwired: 7 in, 1 out]
                      }
                    }
                  }
                  event "SW Trigger": Value Change {
                    n161 = event-data() -> ("NewVal"=w386:bool)  [unwired: 1 in]
                    n162 = case shown="True" w386 {
                      tunnel: [_ w391] -> w387
                      tunnel: w384 -> [_ w390]
                      frame False {
                      }
                      frame True {
                        n163 = call "Send Msg Trigger.vi"("Trigger Msg (F)"=TRUE, "PVName"="Send_Software_Trigger_[TRG]_Msg", "PVConnections"=w390) -> ("error out"=w391:errorcluster)  [unwired: 7 in, 1 out]
                      }
                    }
                  }
                  event "Abort Generation": Value Change {
                    n164 = event-data() -> ("NewVal"=w394:bool)  [unwired: 1 in]
                    n165 = case shown="True" w394 {
                      tunnel: [_ w399] -> w395
                      tunnel: w392 -> [_ w398]
                      frame False {
                      }
                      frame True {
                        n166 = call "Send Msg Trigger.vi"("Trigger Msg (F)"=TRUE, "PVName"="Abort_Generation_Msg", "PVConnections"=w398) -> ("error out"=w399:errorcluster)  [unwired: 7 in, 1 out]
                      }
                    }
                  }
                  event "Clear Arbitrary Memory": Value Change {
                    n167 = event-data() -> ("NewVal"=w402:bool)  [unwired: 1 in]
                    n168 = case shown="True" w402 {
                      tunnel: [_ w407] -> w403
                      tunnel: w400 -> [_ w406]
                      frame False {
                      }
                      frame True {
                        n169 = call "Send Msg Trigger.vi"("Trigger Msg (F)"=TRUE, "PVName"="Clear_Arbitrary_Memory_[SEQ]_Msg", "PVConnections"=w406) -> ("error out"=w407:errorcluster)  [unwired: 7 in, 1 out]
                      }
                    }
                  }
                  event "Clear Arbitrary Sequence": Value Change {
                    n170 = event-data() -> ("NewVal"=w410:bool)  [unwired: 1 in]
                    n171 = case shown="True" w410 {
                      tunnel: [_ w415] -> w411
                      tunnel: w408 -> [_ w413]
                      frame False {
                      }
                      frame True {
                        n172 = call "Send Msg Trigger.vi"("Trigger Msg (F)"=TRUE, "PVName"="Clear_Arbitrary_Sequence_[SEQ]_Msg", "PVConnections"=w413) -> ("error out"=w415:errorcluster)  [unwired: 7 in, 1 out]
                      }
                    }
                  }
                  event "Clear Arbitrary Waveform": Value Change {
                    n173 = event-data() -> ("NewVal"=w418:bool)  [unwired: 1 in]
                    n174 = case shown="True" w418 {
                      tunnel: [_ w423] -> w419
                      tunnel: w416 -> [_ w422]
                      frame False {
                      }
                      frame True {
                        n175 = call "Send Msg Trigger.vi"("Trigger Msg (F)"=TRUE, "PVName"="Clear_Arbitrary_Waveform_[ARB]_Msg", "PVConnections"=w422) -> ("error out"=w423:errorcluster)  [unwired: 7 in, 1 out]
                      }
                    }
                  }
                  event "Sample Clock Output Enabled (Disabled)": Value Change {
                    n176 = event-data() -> ("NewVal"=w427:bool)  [unwired: 1 in]
                    n177 = call "Send Set-Value.vi"("Data"=w427, "PVName"="Configure_Sample_Clock_Output_Enabled_[SC]_Msg", "PVConnections"=w426) -> ("error out"=w424:errorcluster)  [unwired: 7 in, 1 out]
                  }
                  event "Config AM Modulation": Value Change {
                    n178 = event-data() -> ()  [unwired: 1 in, 1 out]
                    n179 = Bundle("AM Modulation Waveform"="AM Modulation Waveform", "modulation depth (0.00 %)"="modulation depth (0.00 %)", "modulation frequency (1000 Hz)"="modulation frequency (1000 Hz)") -> (w430:T7)  [unwired: 1 in]
                    n180 = call "Send Set-Value.vi"("Data"=w430, "PVName"="Configure_AM_Internal_[AM]_Msg", "PVConnections"=w434) -> ("error out"=w429:errorcluster)  [unwired: 7 in, 1 out]
                  }
                  event "Config FM Modulation": Value Change {
                    n181 = event-data() -> ()  [unwired: 1 in, 1 out]
                    n182 = Bundle("FM Modulation Waveform"="FM Modulation Waveform", "FM Peak Deviation"="FM Peak Deviation", "FM Modulation Frequency (1000 Hz)"="FM Modulation Frequency (1000 Hz)") -> (w439:T8)  [unwired: 1 in]
                    n183 = call "Send Set-Value.vi"("Data"=w439, "PVName"="Configure_FM_Internal_[FM]_Msg", "PVConnections"=w442) -> ("error out"=w441:errorcluster)  [unwired: 7 in, 1 out]
                  }
                  event "Sample Rate (1000 Samp/s)": Value Change {
                    n184 = event-data() -> ("NewVal"=w448:dbl[unit])  [unwired: 1 in]
                    n185 = call "Send Set-Value.vi"("Data"=w448, "PVName"="Configure_Sample_Rate_[ARB]_Msg", "PVConnections"=w446) -> ("error out"=w447:errorcluster)  [unwired: 7 in, 1 out]
                  }
                  event "Internal Trigger Rate": Value Change {
                    n186 = event-data() -> ("NewVal"=w451:dbl[unit])  [unwired: 1 in]
                    n187 = call "Send Set-Value.vi"("Data"=w451, "PVName"="Configure_Internal_Trigger_Rate_[IT]_Msg", "PVConnections"=w452) -> ("error out"=w453:errorcluster)  [unwired: 7 in, 1 out]
                  }
                  event "Output Mode": Value Change {
                    n188 = event-data() -> ("NewVal"=w457:i32)  [unwired: 1 in]
                    n189 = call "Send Set-Value.vi"("Data"=w457, "PVName"="Configure_Output_Mode_Msg", "PVConnections"=w456) -> ("error out"=w458:errorcluster)  [unwired: 7 in, 1 out]
                  }
                  event "Reference Clock Source": Value Change {
                    n190 = event-data() -> ("NewVal"=w462:i32)  [unwired: 1 in]
                    n191 = call "Send Set-Value.vi"("Data"=w462, "PVName"="Configure_Ref_Clock_Source_Msg", "PVConnections"=w461) -> ("error out"=w463:errorcluster)  [unwired: 7 in, 1 out]
                  }
                  event "Sample Clock Source (Internal)": Value Change {
                    n192 = event-data() -> ("NewVal"=w467:i32)  [unwired: 1 in]
                    n193 = call "Send Set-Value.vi"("Data"=w467, "PVName"="Configure_Sample_Clock_[SC]_Msg", "PVConnections"=w466) -> ("error out"=w468:errorcluster)  [unwired: 7 in, 1 out]
                  }
                  event "Standard-Waveform.Enabled": Value Change {
                    n194 = event-data() -> ("NewVal"=w471:bool)  [unwired: 1 in]
                    n195 = local read "Channel Index"() -> (w476:i32)
                    n196 = Index Array(array=w477, index=w476) -> (element=w472:string)
                    n197 = Bundle("Substring"=w472, "NewVal"=w471) -> (w470:cluster{"Substring":string, "NewVal":bool})  [unwired: 1 in]
                    n198 = call "Send Set-Value.vi"("Data"=w470, "PVName"="Configure_Output_Enable_Msg", "PVConnections"=w473) -> ("error out"=w475:errorcluster)  [unwired: 7 in, 1 out]
                  }
                  event "Standard-Waveform.Operation Mode": Value Change {
                    n199 = event-data() -> ("NewVal"=w479:i32)  [unwired: 1 in]
                    n200 = local read "Channel Index"() -> (w485:i32)
                    n201 = Index Array(array=w486, index=w485) -> (element=w480:string)
                    n202 = Bundle("Substring"=w480, "NewVal"=w479) -> (w481:cluster{"Substring":string, "NewVal":i32})  [unwired: 1 in]
                    n203 = call "Send Set-Value.vi"("Data"=w481, "PVName"="Configure_Output_Mode_Msg", "PVConnections"=w483) -> ("error out"=w484:errorcluster)  [unwired: 7 in, 1 out]
                  }
                  event "Standard-Waveform.Impedance": Value Change {
                    n204 = event-data() -> ("NewVal"=w489:dbl[unit])  [unwired: 1 in]
                    n205 = local read "Channel Index"() -> (w494:i32)
                    n206 = Index Array(array=w495, index=w494) -> (element=w490:string)
                    n207 = Bundle("Substring"=w490, "NewVal"=w489) -> (w488:cluster{"Substring":string, "NewVal":dbl[unit]})  [unwired: 1 in]
                    n208 = call "Send Set-Value.vi"("Data"=w488, "PVName"="Configure_Output_Impedance_Msg", "PVConnections"=w491) -> ("error out"=w493:errorcluster)  [unwired: 7 in, 1 out]
                  }
                  event "Standard-Waveform.Burst Count": Value Change {
                    n209 = event-data() -> ("NewVal"=w498:i32)  [unwired: 1 in]
                    n210 = local read "Channel Index"() -> (w503:i32)
                    n211 = Index Array(array=w504, index=w503) -> (element=w499:string)
                    n212 = Bundle("Substring"=w499, "NewVal"=w498) -> (w497:cluster{"Substring":string, "NewVal":i32})  [unwired: 1 in]
                    n213 = call "Send Set-Value.vi"("Data"=w497, "PVName"="Configure_Burst_Count_[BST]_Msg", "PVConnections"=w500) -> ("error out"=w502:errorcluster)  [unwired: 7 in, 1 out]
                  }
                  event "Standard-Waveform.Trigger Source": Value Change {
                    n214 = event-data() -> ("NewVal"=w507:i32)  [unwired: 1 in]
                    n215 = local read "Channel Index"() -> (w512:i32)
                    n216 = Index Array(array=w513, index=w512) -> (element=w508:string)
                    n217 = Bundle("Substring"=w508, "NewVal"=w507) -> (w506:cluster{"Substring":string, "NewVal":i32})  [unwired: 1 in]
                    n218 = call "Send Set-Value.vi"("Data"=w506, "PVName"="Configure_Trigger_Source_[TRG]_Msg", "PVConnections"=w510) -> ("error out"=w511:errorcluster)  [unwired: 7 in, 1 out]
                  }
                  event "AM-Modulation.Enabled": Value Change {
                    n219 = event-data() -> ("NewVal"=w516:bool)  [unwired: 1 in]
                    n220 = local read "Channel Index"() -> (w521:i32)
                    n221 = Index Array(array=w522, index=w521) -> (element=w517:string)
                    n222 = Bundle("Substring"=w517, "NewVal"=w516) -> (w515:cluster{"Substring":string, "NewVal":bool})  [unwired: 1 in]
                    n223 = call "Send Set-Value.vi"("Data"=w515, "PVName"="Configure_AM_Enabled_[AM]_Msg", "PVConnections"=w519) -> ("error out"=w520:errorcluster)  [unwired: 7 in, 1 out]
                  }
                  event "AM-Modulation.Source": Value Change {
                    n224 = event-data() -> ("NewVal"=w524:i32)  [unwired: 1 in]
                    n225 = local read "Channel Index"() -> (w530:i32)
                    n226 = Index Array(array=w531, index=w530) -> (element=w525:string)
                    n227 = Bundle("Substring"=w525, "NewVal"=w524) -> (w526:cluster{"Substring":string, "NewVal":i32})  [unwired: 1 in]
                    n228 = call "Send Set-Value.vi"("Data"=w526, "PVName"="Configure_AM_Source_[AM]_Msg", "PVConnections"=w527) -> ("error out"=w529:errorcluster)  [unwired: 7 in, 1 out]
                  }
                  event "FM-Modulation.Enabled": Value Change {
                    n229 = event-data() -> ("NewVal"=w533:bool)  [unwired: 1 in]
                    n230 = local read "Channel Index"() -> (w539:i32)
                    n231 = Index Array(array=w540, index=w539) -> (element=w534:string)
                    n232 = Bundle("Substring"=w534, "NewVal"=w533) -> (w535:cluster{"Substring":string, "NewVal":bool})  [unwired: 1 in]
                    n233 = call "Send Set-Value.vi"("Data"=w535, "PVName"="Configure_FM_Enabled_[FM]_Msg", "PVConnections"=w536) -> ("error out"=w538:errorcluster)  [unwired: 7 in, 1 out]
                  }
                  event "FM-Modulation.Source": Value Change {
                    n234 = event-data() -> ("NewVal"=w543:i32)  [unwired: 1 in]
                    n235 = local read "Channel Index"() -> (w548:i32)
                    n236 = Index Array(array=w549, index=w548) -> (element=w544:string)
                    n237 = Bundle("Substring"=w544, "NewVal"=w543) -> (w542:cluster{"Substring":string, "NewVal":i32})  [unwired: 1 in]
                    n238 = call "Send Set-Value.vi"("Data"=w542, "PVName"="Configure_FM_Source_[FM]_Msg", "PVConnections"=w546) -> ("error out"=w547:errorcluster)  [unwired: 7 in, 1 out]
                  }
                  event "Start Trigger": Value Change {
                    n239 = event-data() -> ("NewVal"=w558:T5)  [unwired: 1 in]
                    n240 = local read "Channel Index"() -> (w559:i32)
                    n241 = Unbundle By Name(w558) -> ("Trigger Slope"=w554:i32, "Trigger Source"=w552:string)
                    n242 = Index Array(array=w560, index=w559) -> (element=w553:string)
                    n243 = Bundle("Trigger Slope"=w554, "Substring"=w553, "Trigger Source"=w552) -> (w551:T9)  [unwired: 1 in]
                    n244 = call "Send Set-Value.vi"("Data"=w551, "PVName"="Configure_Start_Trigger_[STT]_Msg", "PVConnections"=w555) -> ("error out"=w557:errorcluster)  [unwired: 7 in, 1 out]
                  }
                  event "Stop Trigger": Value Change {
                    n245 = event-data() -> ("NewVal"=w569:T4)  [unwired: 1 in]
                    n246 = local read "Channel Index"() -> (w570:i32)
                    n247 = Unbundle By Name(w569) -> ("Trigger Slope)"=w565:i32, "Trigger Source"=w563:string)
                    n248 = Index Array(array=w571, index=w570) -> (element=w564:string)
                    n249 = Bundle("Trigger Slope)"=w565, "Substring"=w564, "Trigger Source"=w563) -> (w562:T10)  [unwired: 1 in]
                    n250 = call "Send Set-Value.vi"("Data"=w562, "PVName"="Configure_Stop_Trigger_[SPT]_Msg", "PVConnections"=w567) -> ("error out"=w568:errorcluster)  [unwired: 7 in, 1 out]
                  }
                  event "Resume Trigger": Value Change {
                    n251 = event-data() -> ("NewVal"=w580:T4)  [unwired: 1 in]
                    n252 = local read "Channel Index"() -> (w581:i32)
                    n253 = Unbundle By Name(w580) -> ("Trigger Slope)"=w576:i32, "Trigger Source"=w574:string)
                    n254 = Index Array(array=w582, index=w581) -> (element=w575:string)
                    n255 = Bundle("Trigger Slope)"=w576, "Substring"=w575, "Trigger Source"=w574) -> (w573:T10)  [unwired: 1 in]
                    n256 = call "Send Set-Value.vi"("Data"=w573, "PVName"="Configure_Resume_Trigger_[RT]_Msg", "PVConnections"=w578) -> ("error out"=w579:errorcluster)  [unwired: 7 in, 1 out]
                  }
                  event "Advanced Trigger": Value Change {
                    n257 = event-data() -> ("NewVal"=w591:T4)  [unwired: 1 in]
                    n258 = local read "Channel Index"() -> (w592:i32)
                    n259 = Unbundle By Name(w591) -> ("Trigger Slope)"=w586:i32, "Trigger Source"=w584:string)
                    n260 = Index Array(array=w593, index=w592) -> (element=w585:string)
                    n261 = Bundle("Trigger Slope)"=w586, "Substring"=w585, "Trigger Source"=w584) -> (w587:T10)  [unwired: 1 in]
                    n262 = call "Send Set-Value.vi"("Data"=w587, "PVName"="Configure_Advanced_Trigger_[AT]_Msg", "PVConnections"=w588) -> ("error out"=w590:errorcluster)  [unwired: 7 in, 1 out]
                  }
                  event "Standard-Waveform.Set/Single", "Standard-Waveform.Start Phase", "Standard-Waveform.Frequency", "Standard-Waveform.DC Offset", "Standard-Waveform.Amplitude", "Standard-Waveform.Waveform": Value Change {
                    n263 = event-data() -> ()  [unwired: 1 in, 3 out]
                    n264 = local read "Channel Index"() -> (w597:i32)
                    n265 = Index Array(array=w609, index=w597) -> (element=w608:string)
                    n266 = Unbundle By Name("Standard-Waveform") -> ("Set/Single"=w598:bool, "Start Phase"=w605:dbl[unit], "Frequency"=w604:dbl[unit], "DC Offset"=w603:dbl[unit], "Amplitude"=w602:dbl[unit], "Waveform"=w601:i32)
                    n267 = call "Write Element of Set_Single.vi"("Set/Single"=w598, "index"=w597, "CS++FgenChannelData in"=w600) -> ("CS++FgenChannelData out"=w599:refnum<class "CS++FgenChannelData.lvclass">)  [unwired: 7 in, 1 out]
                    n268 = case shown="True" w598 {
                      tunnel: w608 -> [_ w612]
                      tunnel: [_ w619] -> w607
                      tunnel: w605 -> [_ w615]
                      tunnel: w604 -> [_ w614]
                      tunnel: w603 -> [_ w613]
                      tunnel: w602 -> [_ w611]
                      tunnel: w601 -> [_ w610]
                      tunnel: "Configure_Standard_Waveform_[STD]_Msg" -> [_ w618]
                      tunnel: w595 -> [_ w617]
                      frame False {
                      }
                      frame True {
                        n269 = Bundle("Start Phase"=w615, "Frequency"=w614, "DC Offset"=w613, "Substring"=w612, "Amplitude"=w611, "Waveform"=w610) -> (w616:T11)  [unwired: 1 in]
                        n270 = call "Send Set-Value.vi"("Data"=w616, "PVName"=w618, "PVConnections"=w617) -> ("error out"=w619:errorcluster)  [unwired: 7 in, 1 out]
                      }
                    }
                  }
                }
                n271 = call <vilib>:"Simple Error Handler.vi"("error in (no error)"=w85) -> ()  [unwired: 4 in, 5 out]
              }
              n272 = Unregister For Events(event registration refnum=w78) -> (error out=w77:errorcluster)  [unwired: 1 in]
              n273 = call-dynamic "Destroy User Define Events.vi"("error in (no error)"=w77, "CS++GUIActor in"=w75) -> ()  [unwired: 8 in, 2 out]
            }
            frame #2 {
              n274 = for {
                tunnel: w620 -> [w623] mode=indexing
                n275 = call "Disconnect.vi"("PVConnection in"=w623) -> ()  [unwired: 9 in, 2 out]
              }
              n276 = call "Open Actor Core FP.vi"("Open FP (F)"=FALSE, "CS++BaseActor in"=w622) -> ()  [unwired: 8 in, 2 out]
            }
          }
        }
        frame Error {
        }
      }
    }
  }
  n277 = call-parent "Actor Core.vi"("error in"=w7, "CS++DeviceGUIActor.lvclass"=w8) -> ("Error Out"=→"Error Out":errorcluster, "Actor out"=→"Actor out":refnum<class "Actor.lvclass">)  [unwired: 8 in]
  n278 = local write "Tab Control 3"(T2."General" ("Tab Control 3")) -> ()
  n279 = local write "Tab Control 2"(enum32{"General", "Channel"}."Channel" ("Tab Control 2")) -> ()
  n280 = local write "Tab Control"(T1."Configuration" ("Tab Control")) -> ()
